vi "ma_SML RT Baseband Zoom FFT.vi"   [LabVIEW 2020, in "NI_MAPro.lvlib"]
uses:
  NI_MAPro.lvlib
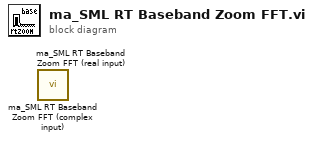
[diagram p0: block diagram]
diagram:
  n1 = call "ma_SML RT Baseband Zoom FFT (complex input).vi"() -> ()  [unwired: 10 in, 6 out]
  n2 = call "ma_SML RT Baseband Zoom FFT (real input).vi"() -> ()  [unwired: 10 in, 6 out]
